vi "PID_Control_de_Posicion_Encoder.vi"() -> ()   [LabVIEW 2025]
uses:
  <vilib>/addons/control/pid/pid.llb/PID (DBL).vi
  <vilib>/addons/control/pid/NI_PID_pid.lvlib
panel:
  in  "output range":cluster{"output high":dbl, "output low":dbl}={"output high"=50.0, "output low"=-100.0} {"output low" format="%.2f"; "output high" format="%.2f"}
  out "output PID":dbl format="%.2f"
  in  "stop":bool
  out "Conteo":dbl
  in  "Restablecer conteo":bool
  in  "Pulsos por revolución":dbl
  out "B":bool
  out "A":bool
  out "Square":dynamicdata(graph)
  out "IN4":bool
  out "IN3":bool
  in  "PID gains":T1={"proportional gain (Kc)"=1.0, "integral time (Ti, min)"=0.01, "derivative time (Td, min)"=0.0} {"derivative time (Td, min)" format="%.3f"; "integral time (Ti, min)" format="%.3f"; "proportional gain (Kc)" format="%.3f"}
  out "Error":dbl
  in  "Setpoint":dbl min=0.0 max=360.0
  out "Posición":dbl(knob) scale=0.0..360.0
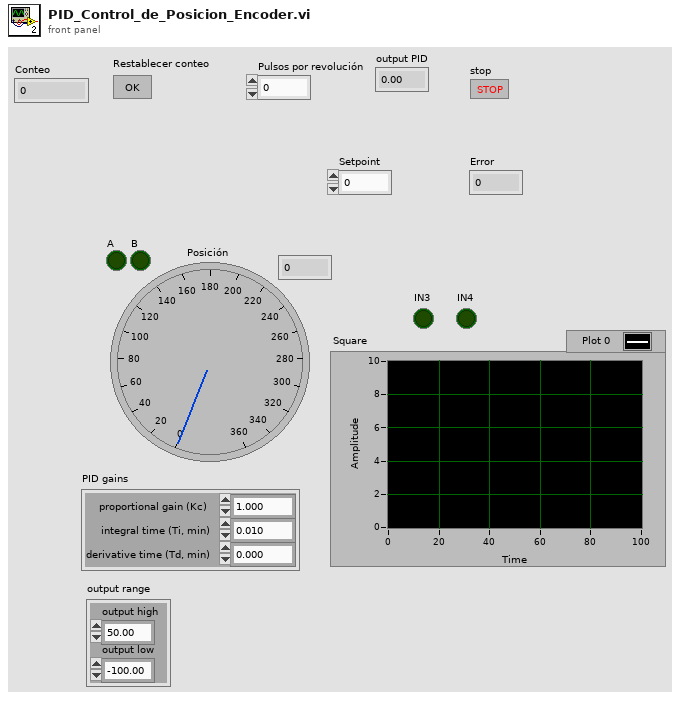
[diagram p1: front panel]
types:
  T1 = cluster{"proportional gain (Kc)":dbl, "integral time (Ti, min)":dbl, "derivative time (Td, min)":dbl}
  T2 = enum16{"Inicio", "L1", "L2", "L3", "Restar", "R1", "R2", "R3", "Sumar", ""}
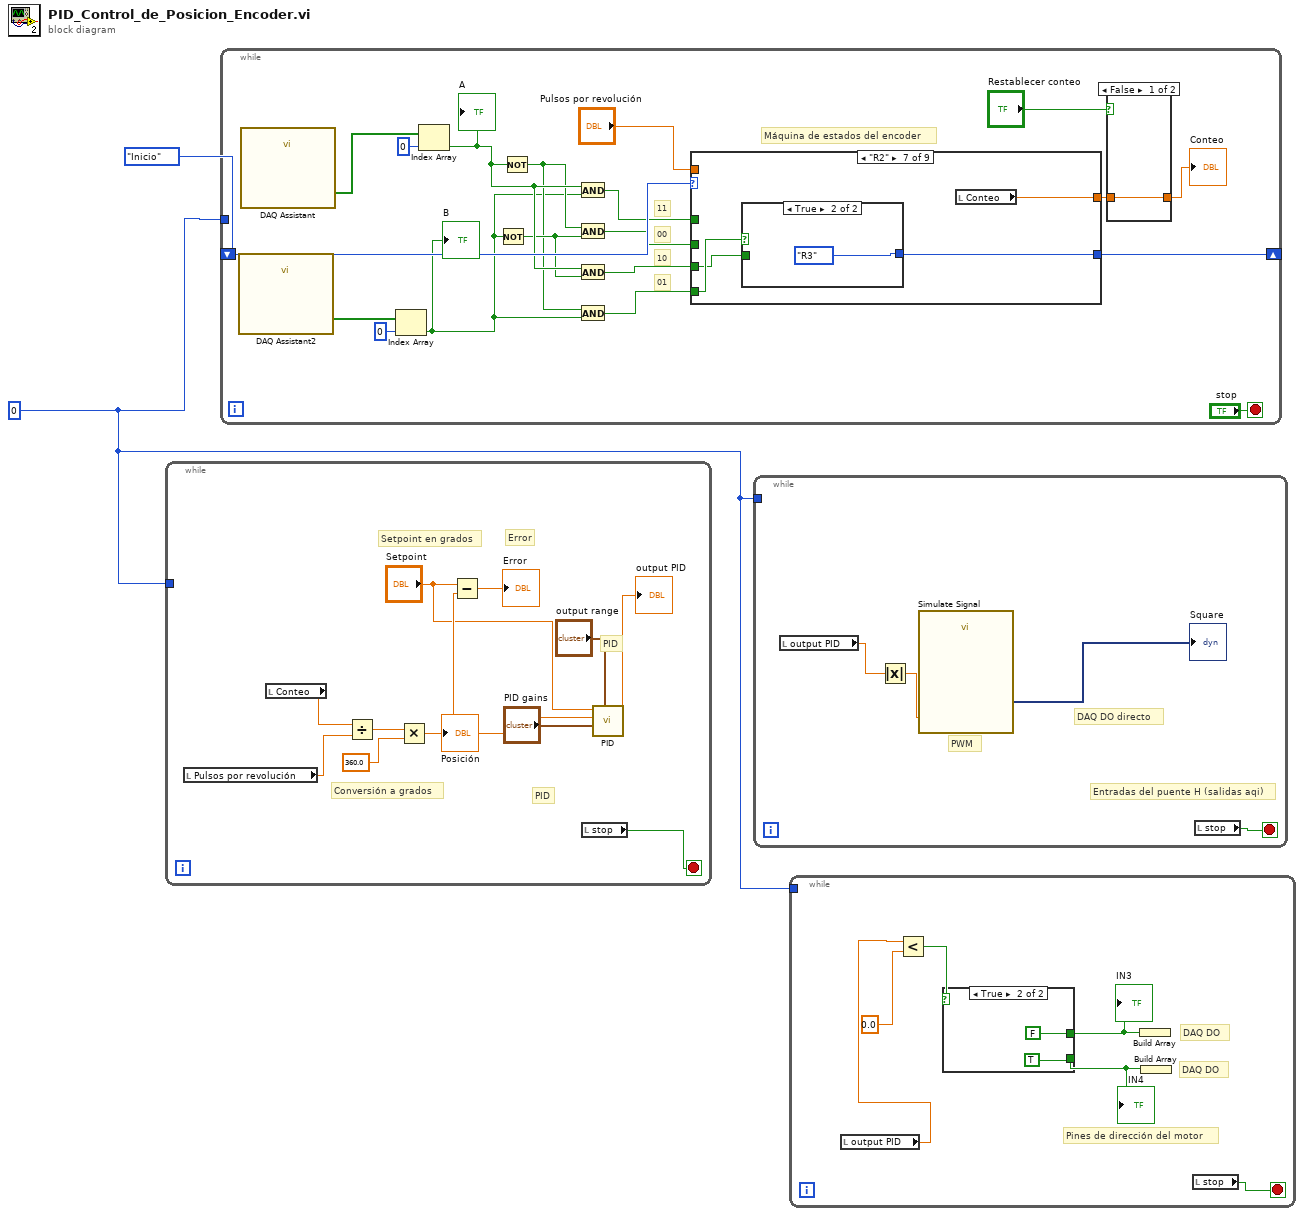
[diagram p0: block diagram]
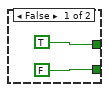
[diagram p2: hidden frame]
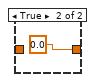
[diagram p3: hidden frame]
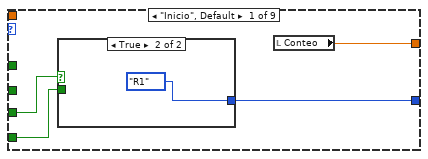
[diagram p4: hidden frame]
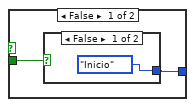
[diagram p5: hidden frame]
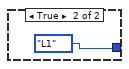
[diagram p6: hidden frame]
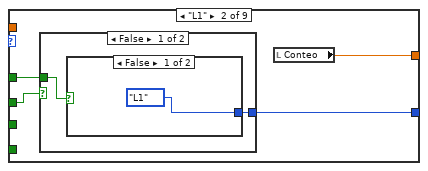
[diagram p7: hidden frame]
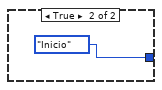
[diagram p8: hidden frame]
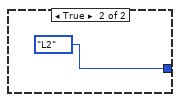
[diagram p9: hidden frame]
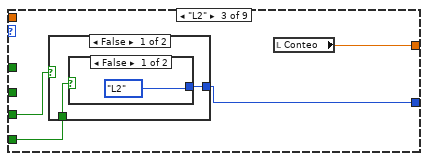
[diagram p10: hidden frame]
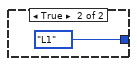
[diagram p11: hidden frame]
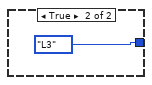
[diagram p12: hidden frame]
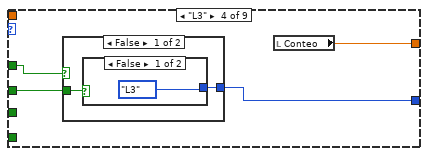
[diagram p13: hidden frame]
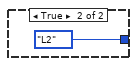
[diagram p14: hidden frame]
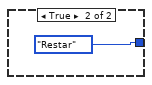
[diagram p15: hidden frame]
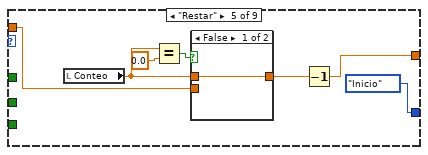
[diagram p16: hidden frame]
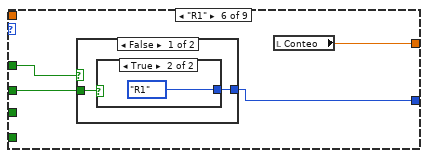
[diagram p18: hidden frame]
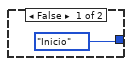
[diagram p19: hidden frame]
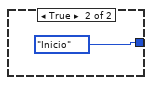
[diagram p20: hidden frame]
diagram:
  w1 = 0
  n1 = while {
    tunnel: w1 -> [_]
    stop <- w3 stop-if-true
    # "PID"
    # "PID"
    # "Error"
    # "Setpoint en grados"
    # "Conversión a grados"
    n2 = local read "Pulsos por revolución"() -> (w13:dbl)
    n3 = local read "Conteo"() -> (w5:dbl)
    n4 = Divide(x=w5, y=w13) -> (x/y=w7:dbl)
    n5 = Multiply(x=w7, y=360.0) -> (x*y=w11:dbl)
    "Posición" <- w11
    n6 = Subtract(x="Setpoint", y=w11) -> (x-y=→"Error":dbl)
    n7 = local read "stop"() -> (w3:bool)
    n8 = call-poly <vilib>:"PID.vi"("output range"="output range", "PID gains"="PID gains", "process variable"=w11, "setpoint"="Setpoint") -> ("output"=→"output PID":dbl)  [unwired: 6 in, 1 out]
  }
  n9 = while {
    shift-right: [w14] -> _
    shift-left: T2."Inicio" -> [w32]
    tunnel: w1 -> [_]
    stop <- "stop" stop-if-true
    # "01"
    # "10"
    # "00"
    # "11"
    # "Máquina de estados del encoder"
    n10 = call "DAQ Assistant2"() -> ("data"=w23:bool[])  [unwired: 17 in, 2 out]
    n11 = call "DAQ Assistant"() -> ("data"=w24:bool[])  [unwired: 17 in, 2 out]
    n12 = Index Array(array=w23, index=0) -> (element=w16:bool)
    "B" <- w16
    n13 = Index Array(array=w24, index=0) -> (element=w20:bool)
    "A" <- w20
    n14 = Not(x=w16) -> (.not. x?=w19:bool)
    n15 = Not(x=w20) -> (.not. x?=w17:bool)
    n16 = And(x=w20, y=w16) -> (x .and. y?=w22:bool)
    n17 = And(x=w17, y=w19) -> (x .and. y?=w21:bool)
    n18 = And(x=w20, y=w19) -> (x .and. y?=w18:bool)
    n19 = And(x=w17, y=w16) -> (x .and. y?=w15:bool)
    n20 = case shown="\"R2\"" w32 {
      tunnel: [w38 w47 w56 w65 w77 w83 w92 w101 w109] -> w29
      tunnel: "Pulsos por revolución" -> [_ _ _ _ w73 _ _ _ w111]
      tunnel: w22 -> [_ w44 _ w63 _ w81 _ w100 _]
      tunnel: w21 -> [_ w45 _ w62 _ w80 _ w99 _]
      tunnel: w18 -> [w37 _ w55 _ _ _ w90 _ _]
      tunnel: w15 -> [w35 _ w54 _ _ _ w91 _ _]
      tunnel: [w36 w46 w53 w64 T2."Inicio" w82 w89 w98 T2."Inicio"] -> w14
      frame "Inicio", Default {
        n21 = case shown="True" w37 {
          tunnel: [w39 T2."R1"] -> w36
          tunnel: w35 -> [w40 _]
          frame False {
            n22 = case shown="False" w40 {
              tunnel: [T2."Inicio" T2."L1"] -> w39
              frame False {
              }
              frame True {
              }
            }
          }
          frame True {
          }
        }
        n23 = local read "Conteo"() -> (w38:dbl)
      }
      frame "L1" {
        n24 = case shown="False" w45 {
          tunnel: [w49 T2."L2"] -> w46
          tunnel: w44 -> [w48 _]
          frame False {
            n25 = case shown="False" w48 {
              tunnel: [T2."L1" T2."Inicio"] -> w49
              frame False {
              }
              frame True {
              }
            }
          }
          frame True {
          }
        }
        n26 = local read "Conteo"() -> (w47:dbl)
      }
      frame "L2" {
        n27 = case shown="False" w55 {
          tunnel: [w58 T2."L3"] -> w53
          tunnel: w54 -> [w57 _]
          frame False {
            n28 = case shown="False" w57 {
              tunnel: [T2."L2" T2."L1"] -> w58
              frame False {
              }
              frame True {
              }
            }
          }
          frame True {
          }
        }
        n29 = local read "Conteo"() -> (w56:dbl)
      }
      frame "L3" {
        n30 = case shown="False" w63 {
          tunnel: [w67 T2."Restar"] -> w64
          tunnel: w62 -> [w66 _]
          frame False {
            n31 = case shown="False" w66 {
              tunnel: [T2."L3" T2."L2"] -> w67
              frame False {
              }
              frame True {
              }
            }
          }
          frame True {
          }
        }
        n32 = local read "Conteo"() -> (w65:dbl)
      }
      frame "Restar" {
        n33 = local read "Conteo"() -> (w72:dbl)
        n34 = Equal?(x=w72, y=0.0) -> (x = y?=w75:bool)
        n35 = case shown="False" w75 {
          tunnel: [w78 w79] -> w74
          tunnel: w73 -> [_ w79]
          tunnel: w72 -> [w78 _]
          frame False {
          }
          frame True {
          }
        }
        n36 = Decrement(x=w74) -> (x-1=w77:dbl)
      }
      frame "R1" {
        n37 = case shown="False" w81 {
          tunnel: [w85 T2."Inicio"] -> w82
          tunnel: w80 -> [w84 _]
          frame False {
            n38 = case shown="True" w84 {
              tunnel: [T2."Inicio" T2."R1"] -> w85
              frame False {
              }
              frame True {
              }
            }
          }
          frame True {
          }
        }
        n39 = local read "Conteo"() -> (w83:dbl)
      }
      frame "R2" {
        n40 = case shown="True" w91 {
          tunnel: [w94 T2."R3"] -> w89
          tunnel: w90 -> [w93 _]
          frame False {
            n41 = case shown="True" w93 {
              tunnel: [T2."R2" T2."R1"] -> w94
              frame False {
              }
              frame True {
              }
            }
          }
          frame True {
          }
        }
        n42 = local read "Conteo"() -> (w92:dbl)
      }
      frame "R3" {
        n43 = case shown="False" w100 {
          tunnel: [w103 T2."Sumar"] -> w98
          tunnel: w99 -> [w102 _]
          frame False {
            n44 = case shown="False" w102 {
              tunnel: [T2."R3" T2."R2"] -> w103
              frame False {
              }
              frame True {
              }
            }
          }
          frame True {
          }
        }
        n45 = local read "Conteo"() -> (w101:dbl)
      }
      frame "Sumar" {
        n46 = local read "Conteo"() -> (w112:dbl)
        n47 = Increment(x=w112) -> (x+1=w108:dbl)
        n48 = Equal?(x=w108, y=w111) -> (x = y?=w110:bool)
        n49 = case shown="True" w110 {
          tunnel: [w113 0.0] -> w109
          tunnel: w108 -> [w113 _]
          frame False {
          }
          frame True {
          }
        }
      }
    }
    n50 = case shown="False" "Restablecer conteo" {
      tunnel: [w33 0.0 ("Conteo")] -> w28
      tunnel: w29 -> [w33 _]
      frame False {
      }
      frame True {
      }
    }
    "Conteo" <- w28
  }
  n51 = while {
    tunnel: w1 -> [_]
    stop <- w115 stop-if-true
    # "DAQ DO directo"
    # "PWM"
    # "Entradas del puente H (salidas aqi)"
    n52 = local read "output PID"() -> (w116:dbl)
    n53 = Absolute Value(x=w116) -> (abs(x)=w118:dbl)
    n54 = call "Simulate Signal"("Duty Cycle (%)"=w118) -> ("Square"=→"Square":dynamicdata)  [unwired: 13 in, 1 out]
    n55 = local read "stop"() -> (w115:bool)
  }
  n56 = while {
    tunnel: w1 -> [_]
    stop <- w119 stop-if-true
    # "DAQ DO"
    # "DAQ DO"
    # "Pines de dirección del motor"
    n57 = local read "output PID"() -> (w120:dbl)
    n58 = Less?(x=w120, y=0.0) -> (x < y?=w122:bool)
    n59 = case shown="True" w122 {
      tunnel: [FALSE TRUE ("IN4")] -> w124
      tunnel: [TRUE FALSE ("IN3")] -> w123
      frame False {
      }
      frame True {
      }
    }
    "IN3" <- w123
    "IN4" <- w124
    n60 = Build Array(w123) -> ()  [unwired: 1 out]
    n61 = Build Array(w124) -> ()  [unwired: 1 out]
    n62 = local read "stop"() -> (w119:bool)
  }
